vi "read_subtable_item.vi"(7 "subtables":string[](array[string]), 8 "error in (no error)":errorcluster, 10 "subkeys":string[](array[string]), 11 "toml in":refnum<class "toml.lvclass">) -> (0 "error out":errorcluster, 1 "found?":bool, 2 "item (value)":refnum<class "Item.lvclass">, 3 "toml out":refnum<class "toml.lvclass">)   [LabVIEW 2020, in "toml.lvclass"]
uses:
  toml.lvclass
  toml.lvclass/toml.ctl
  Item/Item.lvclass
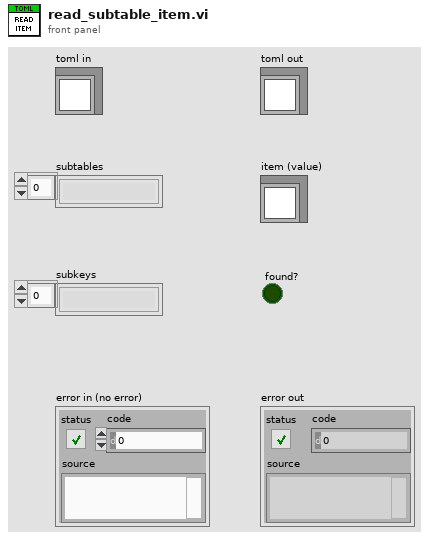
[diagram p1: front panel]
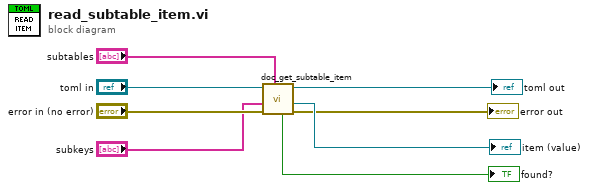
[diagram p0: block diagram]
diagram:
  n1 = call "doc_get_subtable_item.vi"("subtables"="subtables", "error in (no error)"="error in (no error)", "subkeys"="subkeys", "toml in"="toml in") -> ("error out"=→"error out":errorcluster, "item (value)"=→"item (value)":refnum<class "Item.lvclass">, "toml out"=→"toml out":refnum<class "toml.lvclass">, "found?"=→"found?":bool)  [unwired: 4 in]
